vi "Concatenate_and_SetWaveforms.vi"(8 "error in (no error)":errorcluster, 10 "AO Array":waveform(dbl)[](array[waveform]), 11 "DAQ (AO)":refnum<class "DAQ.lvclass">[](array[class])) -> (0 "error out":errorcluster, 2 "AO Array":waveform(dbl)[](array[waveform]), 3 "DAQ (AO)":refnum<class "DAQ.lvclass">[](array[class]))   [LabVIEW 2020, in "DAQ_Manager.lvclass"]
uses:
  DAQ_Manager.lvclass
  DAQ/DAQ.lvclass
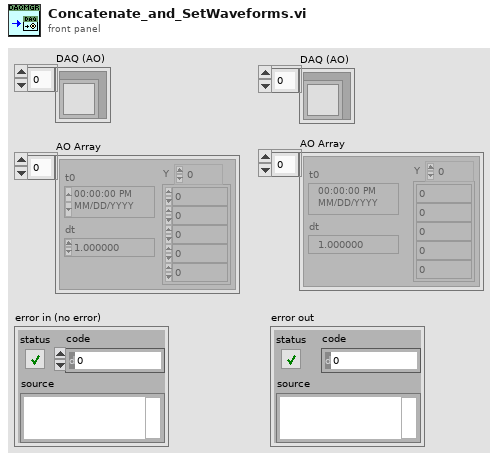
[diagram p1: front panel]
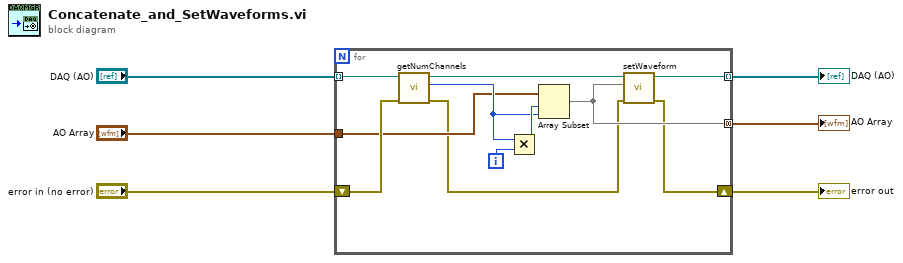
[diagram p0: block diagram]
diagram:
  n1 = for {
    tunnel: [w9] -> w4 mode=concatenating
    shift-right: [w7] -> w3
    shift-left: "error in (no error)" -> [w12]
    tunnel: "AO Array" -> [w10]
    tunnel: "DAQ (AO)" -> [w15] mode=indexing
    tunnel: [w14] -> w2 mode=indexing
    i -> [w16]
    n2 = call "getNumChannels.vi"("error in (no error)"=w12, "DAQ in"=w15) -> ("error out"=w8:errorcluster, "NumChannels"=w13:i32, "DAQ out"=w11:refnum<class "DAQ.lvclass">)  [unwired: 7 in]
    n3 = Multiply(x=w13, y=w16) -> (x*y=w17:i32)
    n4 = Array Subset(array=w10, index=w17, length=w13) -> (w9:waveform(dbl)[])
    n5 = call "setWaveform.vi"("error in (no error)"=w8, "setWaveform"=w9, "DAQ"=w11) -> ("error out"=w7:errorcluster, "DAQ out"=w14:refnum<class "DAQ.lvclass">)  [unwired: 7 in]
  }
  "DAQ (AO)" <- w2
  "AO Array" <- w4
  "error out" <- w3
